vi "resistivity.vi"() -> ()   [LabVIEW 2017]
uses:
  <instrlib>/Keithley 6517/Keithley 6517.lvlib
panel:
  out "resistivity":i32 format="%.6f"
  out "units 2":string
  out "time stamp and date 2":string
  out "reading 2":dbl
  out "channel 2":dbl
  out "units":string
  out "time stamp and date":string
  out "reading":dbl
  out "channel":dbl
  in  "Aperture Integration Time (1.6667000000E-2 s) 2":dbl=0.016667 format="%.10e"
  in  "Enable Average Filter (F: Disable) 2":bool
  in  "Filter Count (10) 2":i32=10
  in  "Enable Zero Correct (F: Disable) 2":bool
  in  "Reading Option (0: Latest) 2":i32(ring) items=["Latest", "New"]
  in  "Display Resolution (6) 2":dbl=6.0
  in  "Auto Range Value (2.0000000E+2) 2":dbl=200.0 format="%.7e"
  in  "Measurement current (1: current)":i32(ring) items=["Voltage", "Current", "Resistance", "Charge"]
  in  "VISA resource name 2":refnum<visa-resource-name>
  in  "Aperture Integration Time (1.6667000000E-2 s)":dbl=0.016667 format="%.10e"
  in  "Enable Average Filter (F: Disable)":bool
  in  "Filter Count (10)":i32=10
  in  "Enable Zero Correct (F: Disable)":bool
  in  "Reading Option (0: Latest)":i32(ring) items=["Latest", "New"]
  in  "Display Resolution (6)":dbl=6.0
  in  "Auto Range Value (2.0000000E+2)":dbl=200.0 format="%.7e"
  in  "Measurement Function (0: Voltage)":i32(ring) items=["Voltage", "Current", "Resistance", "Charge"]
  in  "VISA resource name":refnum<visa-resource-name>
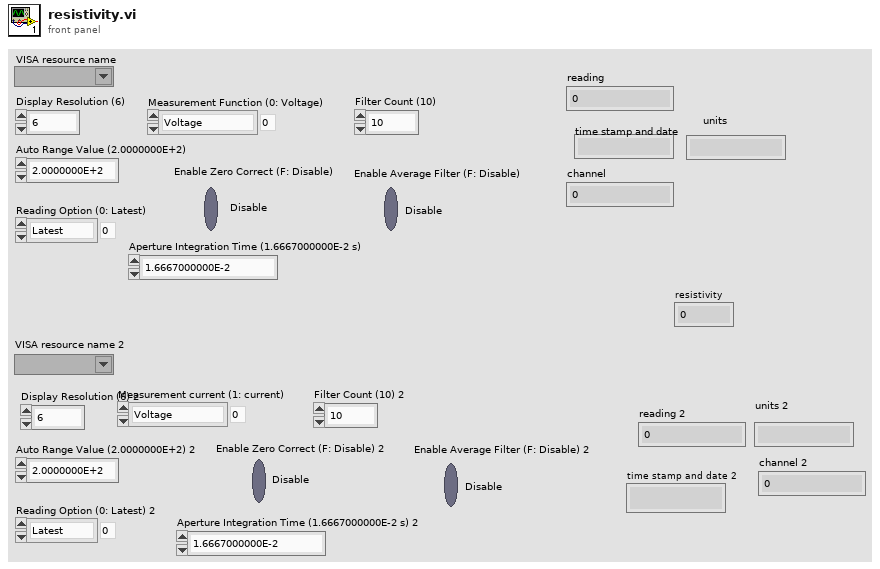
[diagram p1: front panel]
types:
  T1 = cluster{"Measurement":dbl, "Units":string, "Time Stamp and Date":string, "Reading #":dbl, "Channel #":dbl}
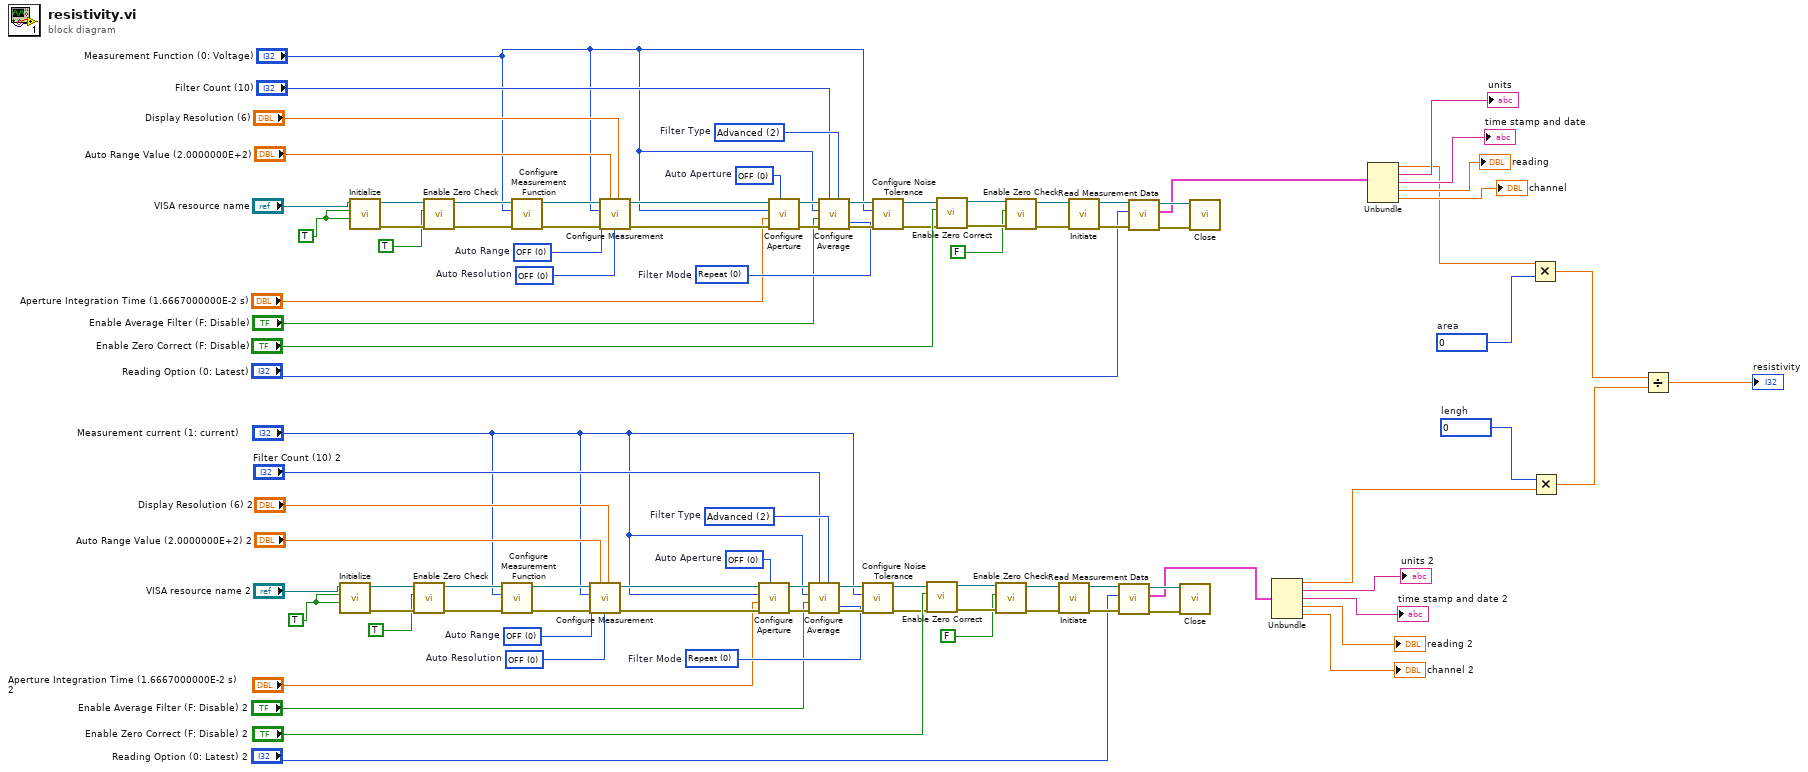
[diagram p0: block diagram]
diagram:
  w11 = 0  # area
  w5 = 0  # lengh
  w27 = 0 items=["OFF", "ON", "ONCE"]  # Auto Aperture
  w24 = 2 items=["None", "Scalar", "Advanced"]  # Filter Type
  w28 = 0 items=["Repeat", "Moving"]  # Filter Mode
  w46 = 0 items=["OFF", "ON", "ONCE"]  # Auto Resolution
  w47 = 0 items=["OFF", "ON", "ONCE"]  # Auto Range
  w55 = TRUE
  w66 = 0 items=["OFF", "ON", "ONCE"]  # Auto Aperture
  w63 = 2 items=["None", "Scalar", "Advanced"]  # Filter Type
  w67 = 0 items=["Repeat", "Moving"]  # Filter Mode
  w85 = 0 items=["OFF", "ON", "ONCE"]  # Auto Resolution
  w86 = 0 items=["OFF", "ON", "ONCE"]  # Auto Range
  w94 = TRUE
  n1 = call <instrlib>:"Initialize.vi"("Reset (True)"=w55, "ID Query (True)"=w55, "VISA resource name"="VISA resource name 2") -> ("error out"=w53:errorcluster, "VISA resource name out"=w54:refnum<visa-resource-name>)  [unwired: 7 in]
  n2 = call <instrlib>:"Initialize.vi"("Reset (True)"=w94, "ID Query (True)"=w94, "VISA resource name"="VISA resource name") -> ("error out"=w92:errorcluster, "VISA resource name out"=w93:refnum<visa-resource-name>)  [unwired: 7 in]
  n3 = call <instrlib>:"Enable Zero Check.vi"("error in (no error)"=w53, "Enable Zero Check (T: Enable)"=TRUE, "VISA resource name"=w54) -> ("error out"=w50:errorcluster, "VISA resource name out"=w51:refnum<visa-resource-name>)  [unwired: 7 in]
  n4 = call <instrlib>:"Enable Zero Check.vi"("error in (no error)"=w92, "Enable Zero Check (T: Enable)"=TRUE, "VISA resource name"=w93) -> ("error out"=w89:errorcluster, "VISA resource name out"=w90:refnum<visa-resource-name>)  [unwired: 7 in]
  n5 = call <instrlib>:"Configure Measurement Function.vi"("error in (no error)"=w50, "Measurement Function (0: Voltage)"="Measurement current (1: current)", "VISA resource name"=w51) -> ("error out"=w48:errorcluster, "VISA resource name out"=w49:refnum<visa-resource-name>)  [unwired: 7 in]
  n6 = call <instrlib>:"Configure Measurement Function.vi"("error in (no error)"=w89, "Measurement Function (0: Voltage)"="Measurement Function (0: Voltage)", "VISA resource name"=w90) -> ("error out"=w87:errorcluster, "VISA resource name out"=w88:refnum<visa-resource-name>)  [unwired: 7 in]
  n7 = call <instrlib>:"Configure Measurement.vi"("Display Resolution (6)"="Display Resolution (6) 2", "Auto Resolution (1: ON)"=w46, "Auto Range Value (2.0000000E+2)"="Auto Range Value (2.0000000E+2) 2", "error in (no error)"=w48, "Auto Range (1: ON)"=w47, "Measurement Function (0: Voltage)"="Measurement current (1: current)", "VISA resource name"=w49) -> ("error out"=w25:errorcluster, "VISA resource name out"=w26:refnum<visa-resource-name>)  [unwired: 3 in]
  n8 = call <instrlib>:"Configure Measurement.vi"("Display Resolution (6)"="Display Resolution (6)", "Auto Resolution (1: ON)"=w85, "Auto Range Value (2.0000000E+2)"="Auto Range Value (2.0000000E+2)", "error in (no error)"=w87, "Auto Range (1: ON)"=w86, "Measurement Function (0: Voltage)"="Measurement Function (0: Voltage)", "VISA resource name"=w88) -> ("error out"=w64:errorcluster, "VISA resource name out"=w65:refnum<visa-resource-name>)  [unwired: 3 in]
  n9 = call <instrlib>:"Configure Aperture.vi"("Auto Aperture (0: OFF)"=w27, "error in (no error)"=w25, "Aperture Integration Time (1.6667000000E-2 s)"="Aperture Integration Time (1.6667000000E-2 s) 2", "Measurement Function (0: Voltage)"="Measurement current (1: current)", "VISA resource name"=w26) -> ("error out"=w29:errorcluster, "VISA resource name out"=w30:refnum<visa-resource-name>)  [unwired: 5 in]
  n10 = call <instrlib>:"Configure Aperture.vi"("Auto Aperture (0: OFF)"=w66, "error in (no error)"=w64, "Aperture Integration Time (1.6667000000E-2 s)"="Aperture Integration Time (1.6667000000E-2 s)", "Measurement Function (0: Voltage)"="Measurement Function (0: Voltage)", "VISA resource name"=w65) -> ("error out"=w68:errorcluster, "VISA resource name out"=w69:refnum<visa-resource-name>)  [unwired: 5 in]
  n11 = call <instrlib>:"Configure Average.vi"("Filter Count (10)"=w24, "Filter Mode (0: Repeat)"=w28, "Filter Type (1: Scalar)"="Filter Count (10) 2", "error in (no error)"=w29, "Enable Average Filter (F: Disable)"="Enable Average Filter (F: Disable) 2", "Measurement Function (0: Voltage)"="Measurement current (1: current)", "VISA resource name"=w30) -> ("error out"=w32:errorcluster, "VISA resource name out"=w31:refnum<visa-resource-name>)  [unwired: 3 in]
  n12 = call <instrlib>:"Configure Average.vi"("Filter Count (10)"=w63, "Filter Mode (0: Repeat)"=w67, "Filter Type (1: Scalar)"="Filter Count (10)", "error in (no error)"=w68, "Enable Average Filter (F: Disable)"="Enable Average Filter (F: Disable)", "Measurement Function (0: Voltage)"="Measurement Function (0: Voltage)", "VISA resource name"=w69) -> ("error out"=w71:errorcluster, "VISA resource name out"=w70:refnum<visa-resource-name>)  [unwired: 3 in]
  n13 = call <instrlib>:"Configure Noise Tolerance.vi"("error in (no error)"=w32, "Measurement Function (0: Voltage)"="Measurement current (1: current)", "VISA resource name"=w31) -> ("error out"=w18:errorcluster, "VISA resource name out"=w19:refnum<visa-resource-name>)  [unwired: 7 in]
  n14 = call <instrlib>:"Configure Noise Tolerance.vi"("error in (no error)"=w71, "Measurement Function (0: Voltage)"="Measurement Function (0: Voltage)", "VISA resource name"=w70) -> ("error out"=w57:errorcluster, "VISA resource name out"=w58:refnum<visa-resource-name>)  [unwired: 7 in]
  n15 = call <instrlib>:"Enable Zero Correct.vi"("error in (no error)"=w18, "Enable Zero Correct (F: Disable)"="Enable Zero Correct (F: Disable) 2", "VISA resource name"=w19) -> ("error out"=w41:errorcluster, "VISA resource name out"=w42:refnum<visa-resource-name>)  [unwired: 7 in]
  n16 = call <instrlib>:"Enable Zero Correct.vi"("error in (no error)"=w57, "Enable Zero Correct (F: Disable)"="Enable Zero Correct (F: Disable)", "VISA resource name"=w58) -> ("error out"=w80:errorcluster, "VISA resource name out"=w81:refnum<visa-resource-name>)  [unwired: 7 in]
  n17 = call <instrlib>:"Enable Zero Check.vi"("error in (no error)"=w41, "Enable Zero Check (T: Enable)"=FALSE, "VISA resource name"=w42) -> ("error out"=w38:errorcluster, "VISA resource name out"=w39:refnum<visa-resource-name>)  [unwired: 7 in]
  n18 = call <instrlib>:"Enable Zero Check.vi"("error in (no error)"=w80, "Enable Zero Check (T: Enable)"=FALSE, "VISA resource name"=w81) -> ("error out"=w77:errorcluster, "VISA resource name out"=w78:refnum<visa-resource-name>)  [unwired: 7 in]
  n19 = call <instrlib>:"Initiate.vi"("error in (no error)"=w38, "VISA resource name"=w39) -> ("error out"=w37:errorcluster, "VISA resource name out"=w36:refnum<visa-resource-name>)  [unwired: 8 in]
  n20 = call <instrlib>:"Initiate.vi"("error in (no error)"=w77, "VISA resource name"=w78) -> ("error out"=w76:errorcluster, "VISA resource name out"=w75:refnum<visa-resource-name>)  [unwired: 8 in]
  n21 = call <instrlib>:"Read Measurement Data.vi"("error in (no error)"=w37, "Reading Option (0: Latest)"="Reading Option (0: Latest) 2", "VISA resource name"=w36) -> ("error out"=w34:errorcluster, "Measurement"=w6:T1, "VISA resource name out"=w33:refnum<visa-resource-name>)  [unwired: 6 in]
  n22 = call <instrlib>:"Read Measurement Data.vi"("error in (no error)"=w76, "Reading Option (0: Latest)"="Reading Option (0: Latest)", "VISA resource name"=w75) -> ("error out"=w73:errorcluster, "Measurement"=w17:T1, "VISA resource name out"=w72:refnum<visa-resource-name>)  [unwired: 6 in]
  n23 = call <instrlib>:"Close.vi"("error in (no error)"=w34, "VISA resource name"=w33) -> ()  [unwired: 9 in, 1 out]
  n24 = call <instrlib>:"Close.vi"("error in (no error)"=w73, "VISA resource name"=w72) -> ()  [unwired: 9 in, 1 out]
  n25 = Unbundle(w6) -> ("Measurement"=w4:dbl, "Units"=→"units 2":string, "Time Stamp and Date"=→"time stamp and date 2":string, "Reading #"=→"reading 2":dbl, "Channel #"=→"channel 2":dbl)
  n26 = Unbundle(w17) -> ("Measurement"=w12:dbl, "Units"=→"units":string, "Time Stamp and Date"=→"time stamp and date":string, "Reading #"=→"reading":dbl, "Channel #"=→"channel":dbl)
  n27 = Multiply(x=w12, y=w11) -> (x*y=w3:dbl)
  n28 = Multiply(x=w5, y=w4) -> (x*y=w2:dbl)
  n29 = Divide(x=w3, y=w2) -> (x/y=→"resistivity":dbl)
